vi "fp button handler_MD.vi"(5 "dummy error input (just for timing purposes)":errorcluster) -> ()   [LabVIEW 2012]
uses:
  <vilib>/Utility/VariantDataType/Type.ctl
  GFG/GFGallGet.vi
  GFG/GFGfpRefGet.vi
  GFG/GFG library.lvlib
  <vilib>/Utility/VariantDataType/VariantType.lvlib
panel:
  out "Source VI":string
  in  "stop":bool
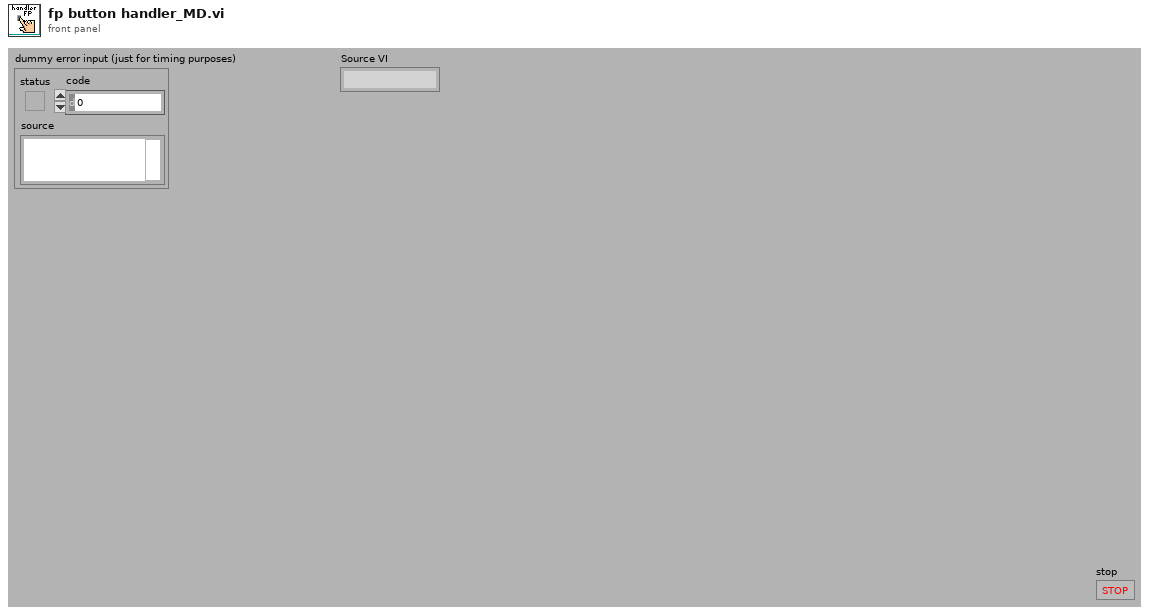
[diagram p1: front panel]
types:
  T1 = typedef "VariantType.lvlib/Type.ctl" = enum8{"Invalid Type", "Void", "I8", "I16", "I32", "I64", "U8", "U16", "U32", "U64", "Single Float", "Double Float", "Extended Float", "Single Complex", "Double Complex", "Extended Complex", "Enum U8", "Enum U16", "Enum U32", "Enum U64", "Single Float With Unit", "Double Float With Unit", "Extended Float With Unit", "Single Complex with Unit", "Double Complex with Unit", "Extended Complex with Unit", "Boolean", "String", "Path", "Picture", "Tag", "Array", "Cluster", "Variant", "LV Variant", "Waveform", "Timestamp", "Digital Waveform", "Digital Data", "ExpressData", "Refnum", "External Data", "VI", "Poly VI", "LabVIEW Class Instance", "Fixed Point"}
  T2 = cluster{"Variable Name Out":string, "Data Type Out":T1, "Variant Out":variant}[]
  T3 = cluster{"WaveformChartRef":refnum<vi>, "DigitalRef":refnum<vi>, "ArrayRef":refnum<vi>, "TabControlRef":refnum<vi>, "EnumRef":refnum<vi>, "RingRef":refnum<vi>, "BooleanRef":refnum<vi>, "KnobRef":refnum<vi>, "SlideRef":refnum<vi>, "PathRef":refnum<vi>, "StringRef":refnum<vi>, "ComboBox":refnum<vi>, "WaveformGraphRef":refnum<vi>}
  T4 = enum8{"Enabled", "Disabled", "Disabled and Grayed Out"}
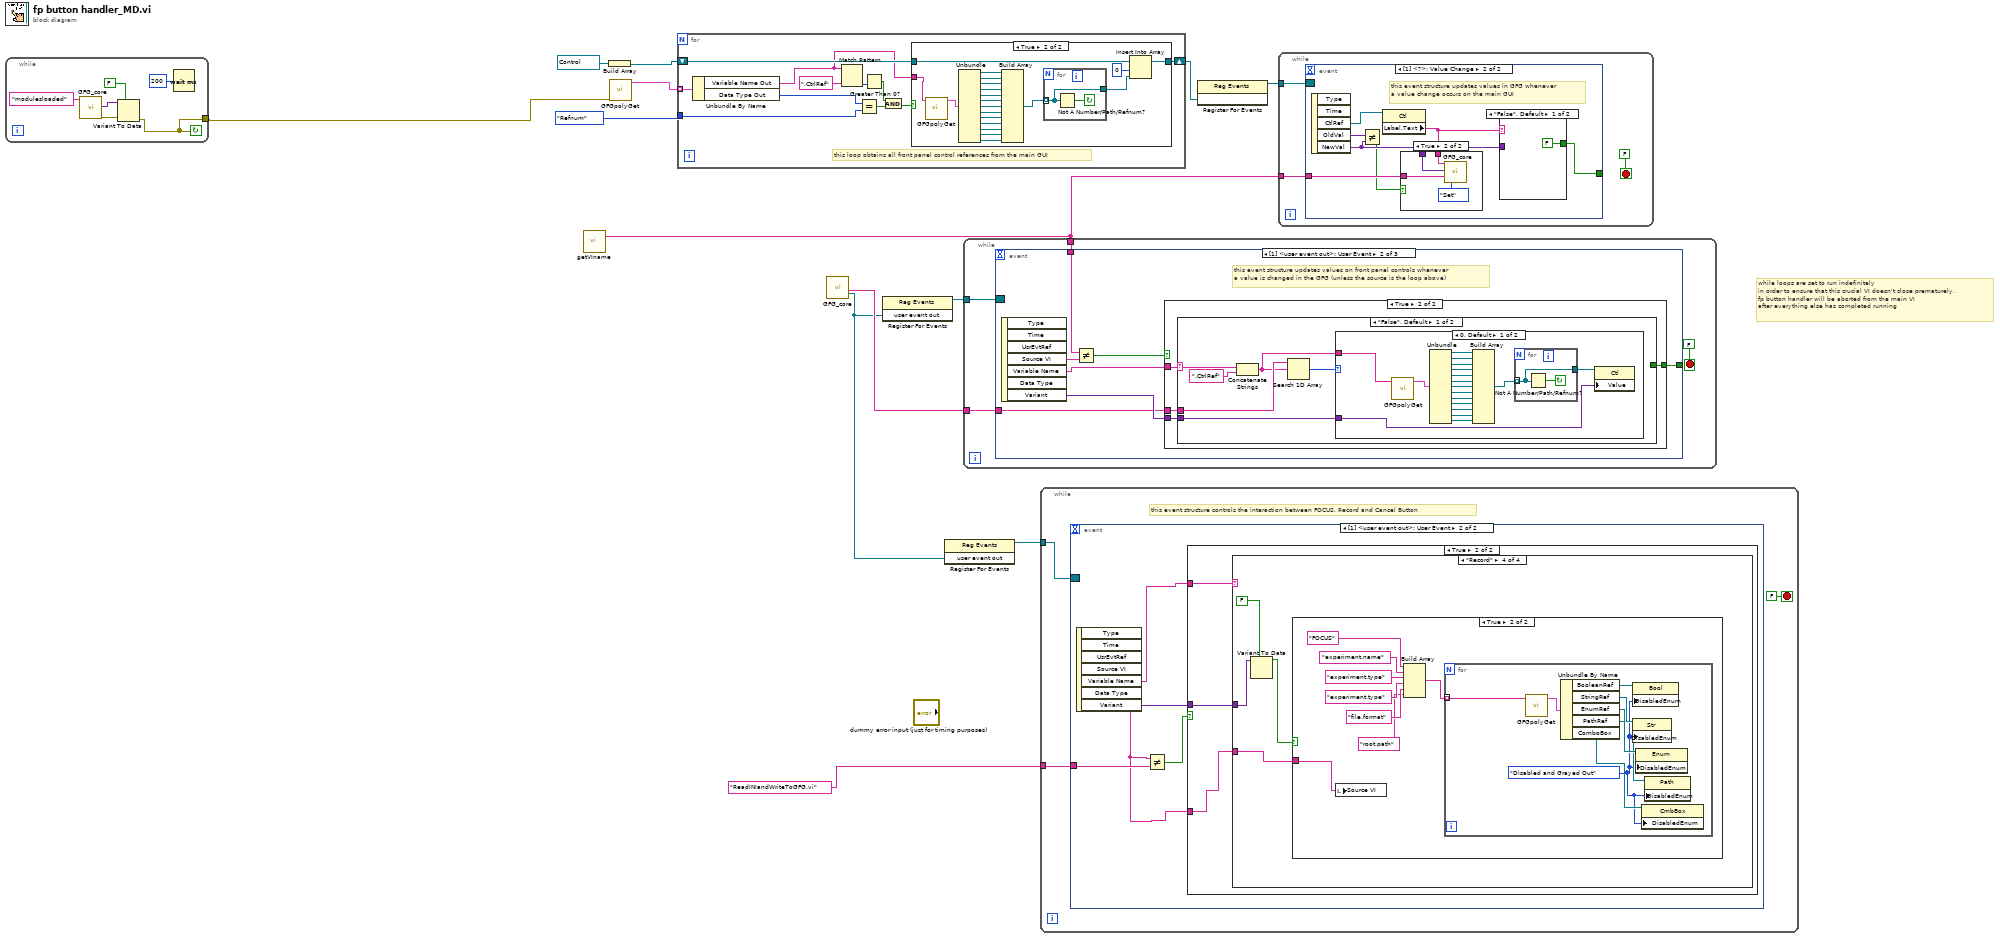
[diagram p0: block diagram]
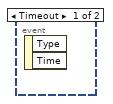
[diagram p2: hidden frame]
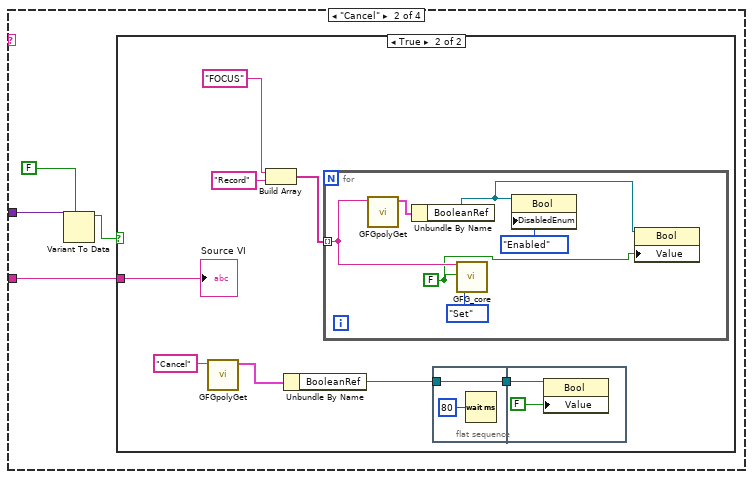
[diagram p5: hidden frame]
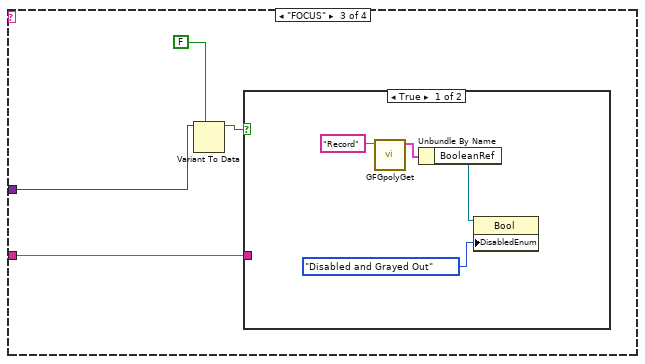
[diagram p7: hidden frame]
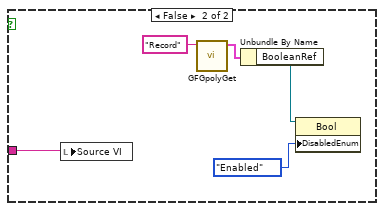
[diagram p8: hidden frame]
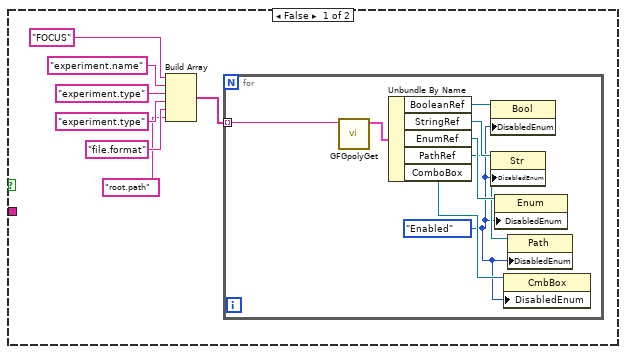
[diagram p9: hidden frame]
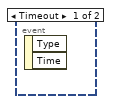
[diagram p10: hidden frame]
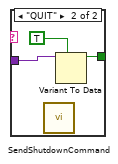
[diagram p12: hidden frame]
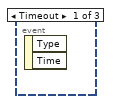
[diagram p14: hidden frame]
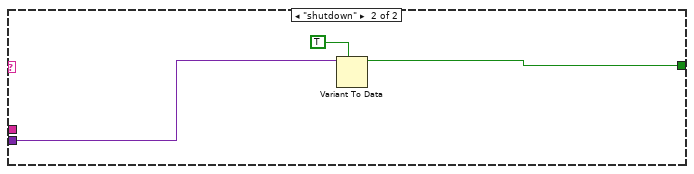
[diagram p17: hidden frame]
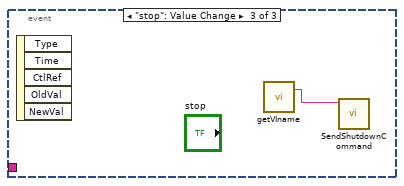
[diagram p18: hidden frame]
diagram:
  # "while loops are set to run indefinitely\nin order to ensure that this crucial VI doesn't close prematurely.\nfp button handler will be aborted from the main VI \nafter everything else has completed running"
  n1 = while {
    tunnel: [w14] -> w1
    stop <- w14 continue-if-true
    n2 = call "GFG_core.vi"("Variable Name in"="modulesloaded") -> ("Variant Out"=w15:variant, "error out"=w17:errorcluster)  [unwired: 12 in, 5 out]
    n3 = Variant To Data(error in=w17, type=FALSE, Variant=w15) -> (error out=w14:errorcluster)  [unwired: 1 out]
    n4 = Wait (ms)(milliseconds to wait=u32 200) -> ()  [unwired: 1 out]
  }
  n5 = call "getVIname.vi"() -> ("VI name"=w5:string)  [unwired: 19 in]
  n6 = Build Array(refnum<vi> refnum ("DigitalRef")) -> (w9:refnum<vi>[])
  n7 = call-poly "GFGpolyGet.vi"("error in (no error)"=w1) -> ("Array of Clusters of Variables"=w11:T2)  [unwired: 9 in, 1 out]
  n8 = for {
    tunnel: w11 -> [w30] mode=indexing
    tunnel: Type."Refnum" ("Data Type Out") -> [w28]
    shift-right: [w26] -> w8
    shift-left: w9 -> [w27]
    # "this loop obtains all front panel control references from the main GUI"
    n9 = Unbundle By Name(w30) -> ("Variable Name Out"=w20:string, "Data Type Out"=w29:T1)
    n10 = Match Pattern(string=w20, regular expression=".CtrlRef" ("string")) -> (offset past match=w24:i32)  [unwired: 1 in, 3 out]
    n11 = Equal?(x=w29, y=w28) -> (x = y?=w21:bool)
    n12 = Greater Than 0?(x=w24) -> (x > 0?=w22:bool)
    n13 = And(x=w22, y=w21) -> (x .and. y?=w23:bool)
    n14 = case shown="True" w23 {
      tunnel: w27 -> [w31 w37]
      tunnel: [w31 w36] -> w26
      tunnel: w20 -> [_ w34]
      frame False {
      }
      frame True {
        n15 = call-poly "GFGpolyGet.vi"("Variable Name in"=w34) -> ("output cluster"=w39:T3)  [unwired: 9 in, 1 out]
        n16 = Unbundle(w39) -> ("WaveformChartRef"=w40:refnum<vi>, "DigitalRef"=w41:refnum<vi>, "ArrayRef"=w42:refnum<vi>, "TabControlRef"=w43:refnum<vi>, "EnumRef"=w44:refnum<vi>, "RingRef"=w45:refnum<vi>, "BooleanRef"=w46:refnum<vi>, "KnobRef"=w47:refnum<vi>, "SlideRef"=w48:refnum<vi>, "PathRef"=w49:refnum<vi>, "StringRef"=w50:refnum<vi>, "ComboBox"=w33:refnum<vi>, "WaveformGraphRef"=w32:refnum<vi>)
        n17 = Build Array(w40, w41, w42, w43, w44, w45, w46, w47, w48, w49, w50, w33, w32) -> (w51:refnum<vi>[])
        n18 = for {
          tunnel: w51 -> [w52] mode=indexing
          tunnel: [w52] -> w38
          stop <- w53 continue-if-true
          n19 = Not A Number/Path/Refnum?(number/path/refnum=w52) -> (NaN/Path/Refnum?=w53:bool)
        }
        n20 = Insert Into Array(array=w37, index=0, new element=w38) -> (w36:refnum<vi>[])
      }
    }
  }
  n21 = call "GFG_core.vi"() -> ("All Variable Names Out"=w12:string[], "user event out"=w3:refnum<user-event>)  [unwired: 13 in, 5 out]
  n22 = register-events(w3) -> (reference out=w13:refnum<event-registration>)  [unwired: 2 in, 1 out]
  n23 = register-events(w3) -> (reference out=w6:refnum<event-registration>)  [unwired: 2 in, 1 out]
  n24 = while {
    tunnel: w13 -> [w57]
    tunnel: w12 -> [w56]
    tunnel: w5 -> [w55]
    stop <- FALSE stop-if-true
    n25 = event shown="[1] <user event out>: User Event" {
      selector: w57 -> [_ _ _]
      dyn-events: _ -> [_ _ _]
      timeout: _ -> [_ _ _]
      tunnel: [_ w62 _] -> _
      tunnel: w56 -> [_ w61 _]
      tunnel: w55 -> [_ w60 _]
      event Timeout {
        n26 = event-data() -> ()  [unwired: 1 in, 2 out]
      }
      event User Event {
        # "this event structure updates values on front panel controls whenever\na value is changed in the GFG (unless the source is the loop above)"
        n27 = event-data() -> ("Source VI"=w59:string, "Variable Name"=w64:string, "Variant"=w63:variant)  [unwired: 1 in, 4 out]
        n28 = Not Equal?(x=w60, y=w59) -> (x != y?=w58:bool)
        n29 = case shown="True" w58 {
          tunnel: w64 -> [_ w68]
          tunnel: w63 -> [_ w67]
          tunnel: [_ w66] -> w62
          tunnel: w61 -> [_ w65]
          frame False {
          }
          frame True {
            n30 = case shown="\"False\", Default" w68 {
              selector: w68 -> [w73 _]
              tunnel: w67 -> [w69 w97]
              tunnel: [_ w95] -> w66
              tunnel: w65 -> [w72 _]
              frame "False", Default {
                n31 = Concatenate Strings(w73, ".CtrlRef" ("string")) -> (w70:string)
                n32 = Search 1D Array(1D array=w72, element=w70) -> (index of element=w71:i32)  [unwired: 1 in]
                n33 = case shown="0, Default" w71 {
                  tunnel: w70 -> [w92 _]
                  tunnel: w69 -> [w77 _]
                  frame 0, Default {
                    n34 = call-poly "GFGpolyGet.vi"("Variable Name in"=w92) -> ("output cluster"=w91:T3)  [unwired: 9 in, 1 out]
                    n35 = Unbundle(w91) -> ("WaveformChartRef"=w90:refnum<vi>, "DigitalRef"=w89:refnum<vi>, "ArrayRef"=w88:refnum<vi>, "TabControlRef"=w87:refnum<vi>, "EnumRef"=w86:refnum<vi>, "RingRef"=w85:refnum<vi>, "BooleanRef"=w84:refnum<vi>, "KnobRef"=w83:refnum<vi>, "SlideRef"=w82:refnum<vi>, "PathRef"=w81:refnum<vi>, "StringRef"=w80:refnum<vi>, "ComboBox"=w76:refnum<vi>, "WaveformGraphRef"=w75:refnum<vi>)
                    n36 = Build Array(w90, w89, w88, w87, w86, w85, w84, w83, w82, w81, w80, w76, w75) -> (w79:refnum<vi>[])
                    n37 = for {
                      tunnel: w79 -> [w93] mode=indexing
                      tunnel: [w93] -> w78
                      stop <- w94 continue-if-true
                      n38 = Not A Number/Path/Refnum?(number/path/refnum=w93) -> (NaN/Path/Refnum?=w94:bool)
                    }
                    n39 = property class="Ctl"(reference=w78, "Value"=w77) -> ()  [unwired: 1 in, 2 out]
                  }
                  frame -1 {
                  }
                }
              }
              frame "shutdown" {
                n40 = Variant To Data(type=TRUE ("want seconds? (F)"), Variant=w97) -> (data=w95:bool)  [unwired: 1 in, 1 out]
              }
            }
          }
        }
      }
      event "stop": Value Change {
        n41 = event-data() -> ()  [unwired: 1 in, 5 out]
        n42 = call "getVIname.vi"() -> ("VI name"=w98:string)  [unwired: 19 in]
        n43 = call "SendShutdownCommand.vi"("Source VI"=w98) -> ()  [unwired: 11 in]
      }
    }
  }
  n44 = while {
    tunnel: w6 -> [w101]
    tunnel: "ReadINIandWriteToGFG.vi" ("Source VI") -> [w99]
    stop <- FALSE stop-if-true
    # "this event structure controls the interaction between FOCUS, Record and Cancel Button"
    n45 = event shown="[1] <user event out>: User Event" {
      selector: w101 -> [_ _]
      dyn-events: _ -> [_ _]
      timeout: _ -> [_ _]
      tunnel: w99 -> [_ w104]
      event Timeout {
        n46 = event-data() -> ()  [unwired: 1 in, 2 out]
      }
      event User Event {
        n47 = event-data() -> ("Source VI"=w102:string, "Variable Name"=w106:string, "Variant"=w105:variant)  [unwired: 1 in, 4 out]
        n48 = Not Equal?(x=w102, y=w104) -> (x != y?=w103:bool)
        n49 = case shown="True" w103 {
          tunnel: w106 -> [_ w109]
          tunnel: w105 -> [_ w108]
          tunnel: w102 -> [_ w107]
          frame False {
          }
          frame True {
            n50 = case shown="\"Record\"" w109 {
              tunnel: w108 -> [_ w113 w134 w148]
              tunnel: w107 -> [_ w110 w132 w145]
              frame "False", Default {
              }
              frame "Cancel" {
                n51 = Variant To Data(type=FALSE, Variant=w113) -> (data=w111:bool)  [unwired: 1 in, 1 out]
                n52 = case shown="True" w111 {
                  tunnel: w110 -> [_ w114]
                  frame False {
                  }
                  frame True {
                    n53 = call-poly "GFGpolyGet.vi"("Variable Name in"="Cancel") -> ("output cluster"=w116:T3)  [unwired: 9 in, 1 out]
                    n54 = Build Array("FOCUS" ("Variable Name in"), "Record" ("element")) -> (w118:string[])
                    n55 = Unbundle By Name(w116) -> ("BooleanRef"=w115:refnum<vi>)
                    n56 = for {
                      tunnel: w118 -> [w128] mode=indexing
                      w126 = FALSE
                      n57 = call-poly "GFGpolyGet.vi"("Variable Name in"=w128) -> ("output cluster"=w130:T3)  [unwired: 9 in, 1 out]
                      n58 = Unbundle By Name(w130) -> ("BooleanRef"=w127:refnum<vi>)
                      n59 = call "GFG_core.vi"("Variable Name in"=w128, "Variant in"=w126, "Action"=enum16{"Init", "Set", "Get"}."Set") -> ()  [unwired: 10 in, 7 out]
                      n60 = property class="Bool"(reference=w127, "DisabledEnum"=T4."Enabled" ("Disabled")) -> ()  [unwired: 1 in, 2 out]
                      n61 = property class="Bool"(reference=w127, "Value"=w126) -> ()  [unwired: 1 in, 2 out]
                    }
                    n62 = flat-sequence {
                      tunnel: w115 -> [w123]
                      tunnel: [w123] -> w121
                      tunnel: w121 -> [w125]
                      frame #0 {
                        n63 = Wait (ms)(milliseconds to wait=u32 80) -> ()  [unwired: 1 out]
                      }
                      frame #1 {
                        n64 = property class="Bool"(reference=w125, "Value"=FALSE) -> ()  [unwired: 1 in, 2 out]
                      }
                    }
                    "Source VI" <- w114
                  }
                }
              }
              frame "FOCUS" {
                n65 = Variant To Data(type=FALSE ("NewVal"), Variant=w134) -> (data=w133:bool)  [unwired: 1 in, 1 out]
                n66 = case shown="True" w133 {
                  tunnel: w132 -> [_ w140]
                  frame True {
                    n67 = call-poly "GFGpolyGet.vi"("Variable Name in"="Record") -> ("output cluster"=w137:T3)  [unwired: 9 in, 1 out]
                    n68 = Unbundle By Name(w137) -> ("BooleanRef"=w136:refnum<vi>)
                    n69 = property class="Bool"(reference=w136, "DisabledEnum"=T4."Disabled and Grayed Out" ("Disabled")) -> ()  [unwired: 1 in, 2 out]
                  }
                  frame False {
                    n70 = local write "Source VI"(w140) -> ()
                    n71 = call-poly "GFGpolyGet.vi"("Variable Name in"="Record") -> ("output cluster"=w142:T3)  [unwired: 9 in, 1 out]
                    n72 = Unbundle By Name(w142) -> ("BooleanRef"=w141:refnum<vi>)
                    n73 = property class="Bool"(reference=w141, "DisabledEnum"=T4."Enabled" ("Disabled")) -> ()  [unwired: 1 in, 2 out]
                  }
                }
              }
              frame "Record" {
                n74 = Variant To Data(type=FALSE ("NewVal"), Variant=w148) -> (data=w146:bool)  [unwired: 1 in, 1 out]
                n75 = case shown="True" w146 {
                  tunnel: w145 -> [_ w164]
                  frame False {
                    n76 = Build Array("FOCUS" ("Variable Name in"), "experiment.name" ("element"), "experiment.type" ("element"), "experiment.type" ("element"), "file.format" ("element"), "root.path" ("element")) -> (w150:string[])
                    n77 = for {
                      tunnel: w150 -> [w161] mode=indexing
                      w156 = T4."Enabled" ("Disabled")
                      n78 = call-poly "GFGpolyGet.vi"("Variable Name in"=w161) -> ("output cluster"=w163:T3)  [unwired: 9 in, 1 out]
                      n79 = Unbundle By Name(w163) -> ("BooleanRef"=w162:refnum<vi>, "StringRef"=w160:refnum<vi>, "EnumRef"=w159:refnum<vi>, "PathRef"=w158:refnum<vi>, "ComboBox"=w157:refnum<vi>)
                      n80 = property class="Bool"(reference=w162, "DisabledEnum"=w156) -> ()  [unwired: 1 in, 2 out]
                      n81 = property class="Str"(reference=w160, "DisabledEnum"=w156) -> ()  [unwired: 1 in, 2 out]
                      n82 = property class="Enum"(reference=w159, "DisabledEnum"=w156) -> ()  [unwired: 1 in, 2 out]
                      n83 = property class="CmbBox"(reference=w157, "DisabledEnum"=w156) -> ()  [unwired: 1 in, 2 out]
                      n84 = property class="Path"(reference=w158, "DisabledEnum"=w156) -> ()  [unwired: 1 in, 2 out]
                    }
                  }
                  frame True {
                    n85 = local write "Source VI"(w164) -> ()
                    n86 = Build Array("FOCUS" ("Variable Name in"), "experiment.name" ("element"), "experiment.type" ("element"), "experiment.type" ("element"), "file.format" ("element"), "root.path" ("element")) -> (w166:string[])
                    n87 = for {
                      tunnel: w166 -> [w177] mode=indexing
                      w172 = T4."Disabled and Grayed Out" ("Disabled")
                      n88 = call-poly "GFGpolyGet.vi"("Variable Name in"=w177) -> ("output cluster"=w179:T3)  [unwired: 9 in, 1 out]
                      n89 = Unbundle By Name(w179) -> ("BooleanRef"=w178:refnum<vi>, "StringRef"=w176:refnum<vi>, "EnumRef"=w175:refnum<vi>, "PathRef"=w174:refnum<vi>, "ComboBox"=w173:refnum<vi>)
                      n90 = property class="Bool"(reference=w178, "DisabledEnum"=w172) -> ()  [unwired: 1 in, 2 out]
                      n91 = property class="Str"(reference=w176, "DisabledEnum"=w172) -> ()  [unwired: 1 in, 2 out]
                      n92 = property class="Enum"(reference=w175, "DisabledEnum"=w172) -> ()  [unwired: 1 in, 2 out]
                      n93 = property class="CmbBox"(reference=w173, "DisabledEnum"=w172) -> ()  [unwired: 1 in, 2 out]
                      n94 = property class="Path"(reference=w174, "DisabledEnum"=w172) -> ()  [unwired: 1 in, 2 out]
                    }
                  }
                }
              }
            }
          }
        }
      }
    }
  }
  n95 = register-events(w8) -> (reference out=w7:refnum<event-registration>)  [unwired: 2 in, 1 out]
  n96 = while {
    tunnel: w7 -> [w182]
    tunnel: w5 -> [w181]
    stop <- FALSE stop-if-true
    n97 = event shown="[1] <?>: Value Change" {
      selector: w182 -> [_ _]
      dyn-events: _ -> [_ _]
      timeout: _ -> [_ _]
      tunnel: w181 -> [_ w188]
      tunnel: [_ w186] -> _
      event Timeout {
        n98 = event-data() -> ()  [unwired: 1 in, 2 out]
      }
      event Value Change {
        # "this event structure updates values in GFG whenever\na value change occurs on the main GUI"
        n99 = event-data() -> ("CtlRef"=w189:refnum<vi>, "OldVal"=w185:variant, "NewVal"=w184:variant)  [unwired: 1 in, 2 out]
        n100 = Not Equal?(x=w185, y=w184) -> (x != y?=w183:bool)
        n101 = property class="Ctl"(reference=w189) -> ("Label.Text"=w187:string)  [unwired: 1 in, 2 out]
        n102 = case shown="True" w183 {
          tunnel: w188 -> [_ w192]
          tunnel: w187 -> [_ w191]
          tunnel: w184 -> [_ w190]
          frame False {
          }
          frame True {
            n103 = call "GFG_core.vi"("Variable Name in"=w191, "Variant in"=w190, "Source VI"=w192, "Action"=enum16{"Init", "Set", "Get"}."Set") -> ()  [unwired: 9 in, 7 out]
          }
        }
        n104 = case shown="\"False\", Default" w187 {
          tunnel: w184 -> [_ w197]
          tunnel: [FALSE w195] -> w186
          frame "False", Default {
          }
          frame "QUIT" {
            n105 = call "SendShutdownCommand.vi"() -> ()  [unwired: 12 in]
            n106 = Variant To Data(type=TRUE, Variant=w197) -> (data=w195:bool)  [unwired: 1 in, 1 out]
          }
        }
      }
    }
  }
